vi "RSZVB Set Virtual Transform Balanced Port.vi"(0 "VISA session":refnum<visa-resource-name>, 1 "Parameter Number (1)":i32=1, 2 "Value (1.0e-12 F  (Capacitance))":dbl=1e-12 format="%^.3e", 5 "Channel (1)":i32=1, 7 "Function Type (0: Deembedding)":i32(ring) items=["Deembedding", "Embedding"], 9 "Logical Port Number (1)":i32=1, 11 "error in (no error)":errorcluster {"code" format="%.0x"}, 12 "Circuit Model (1:Serial Touchstone (.s2p) data, shunt L)":i32(ring)=1 items=["Serial Touchstone (.s2p) data, shunt L"=1, "Serial Touchstone (.s2p) data, shunt C"=2, "Shunt L, serial Touchstone (.s2p) data"=3, "Shunt C, serial Touchstone (.s2p) data"=4, "Serial Cs, shunt L"=5, "Serial Ls, shunt C"=6, "Serial Cs, shunt C"=7, "Serial Ls, shunt L"=8, "Shunt L, serial Cs"=9, "Shunt C, serial Ls"=10, "Shunt C, serial Cs"=11, "Shunt L, serial Ls"=12], 13 "Parameter Type (0: Capacitance)":i32(ring) items=["Capacitance", "Inductance", "Resistance"]) -> (4 "dup VISA session":refnum<visa-resource-name>, 15 "error out":errorcluster {"code" format="%.0x"})   [LabVIEW 2011]
doc: "This VI specifies the capacitance, inductance or resistance values C1, C2, C3, L1, L2, L3 or R1, R2, R3 in the different circuit models for balanced port deembedding/embedding.\n\nRemote-control command(s):\nCALCulate<Ch>:TRANsform:VNETworks:BALanced:DEEMbedding<Log_pt>:PARameters:C<no> STSC | SCST | CSSL | LSSC | CSSC | SLCS | SCLS | SCCS,<numeric_value>\nCALCulate<Ch>:TRANsform:VNETworks:BALanced:DEEMbedding<Log_pt>:PARameters:L<no> STSL | SLST | CSSL | LSSC | LSSL | SLCS | SCLS | SLLS,<numeric_value>\nCALCulate<Ch>:TRANsform:VNETworks:BALanced:DEEMbedding<Log_pt>:PARameters:R<no> STSL | STSC | SLST | SCST | CSSL | LSSC | CSSC | LSSL | SLCS | SCLS | SCCS | SLLS,<numeric_value>\nCALCulate<Ch>:TRANsform:VNETworks:BALanced:EMBedding<Log_pt>:PARameters:C<no> STSC | SCST | CSSL | LSSC | CSSC | SLCS | SCLS | SCCS,<numeric_value>\nCALCulate<Ch>:TRANsform:VNETworks:BALanced:EMBedding<Log_pt>:PARameters:L<no> STSL | SLST | CSSL | LSSC | LSSL | SLCS | SCLS | SLLS,<numeric_value>\nCALCulate<Ch>:TRANsform:VNETworks:BALanced:EMBedding<Log_pt>:PARameters:R<no> STSL | STSC | SLST | SCST | CSSL | LSSC | CSSC | LSSL | SLCS | SCLS | SCCS | SLLS,<numeric_value>"
uses:
  _utility/RSZVB Global Data.vi
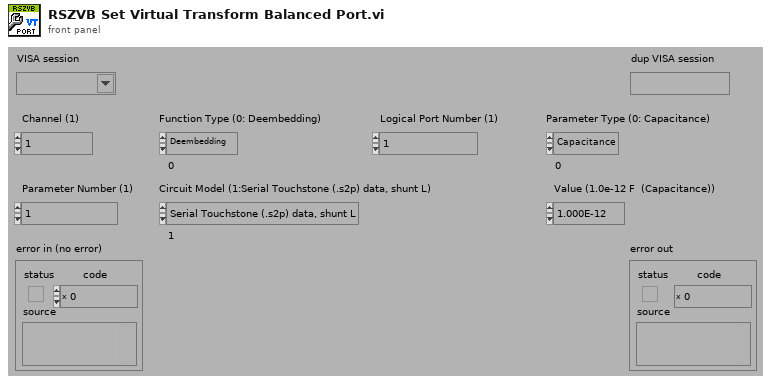
[diagram p1: front panel]
types:
  T1 = cluster{"Error Checking (T: On)":bool, "Installed Options":string[], "Data Valid?":bool, "Ports":i32, "Model":string[], "Option Checking (T: On)":bool}[]
  T2 = cluster{"Error Checking (T: On)":bool, "Installed Options":string[], "Data Valid?":bool, "Ports":i32, "Model":string[], "Option Checking (T: On)":bool}
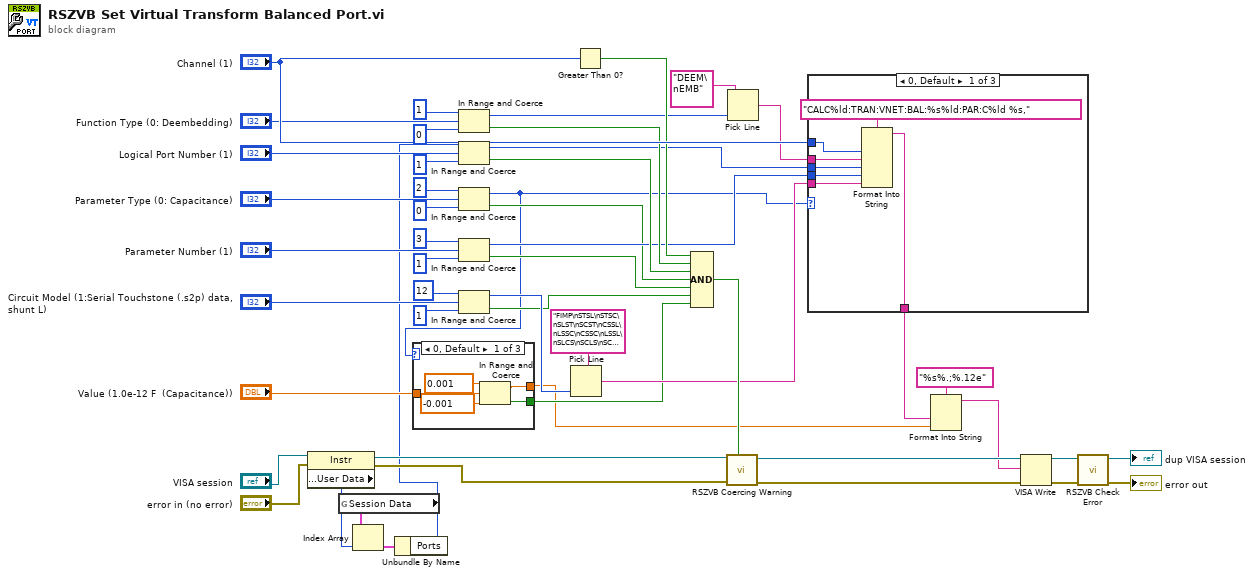
[diagram p0: block diagram]
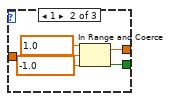
[diagram p2: hidden frame]
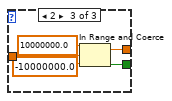
[diagram p3: hidden frame]
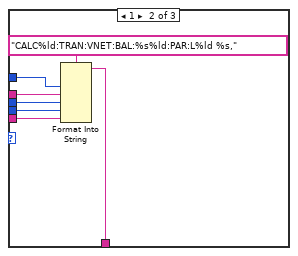
[diagram p4: hidden frame]
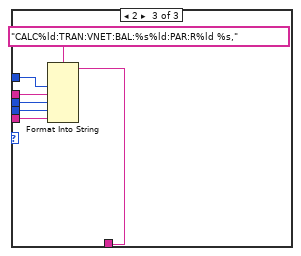
[diagram p5: hidden frame]
diagram:
  n1 = property class="Instr"(reference="VISA session", error in="error in (no error)") -> (reference out=w42:refnum<visa-resource-name>, error out=w43:errorcluster, "General Settings:User Data"=w46:u32)
  n2 = global read "RSZVB Global Data.vi" "Session Data"() -> (w45:T1)
  n3 = Index Array(array=w45, index=w46) -> (element=w44:T2)
  n4 = Unbundle By Name(w44) -> ("Ports"=w1:i32)
  n5 = In Range and Coerce(upper limit=1 ("lower limit"), x="Function Type (0: Deembedding)", lower limit=0) -> (coerced(x)=w33:i32, In Range?=w36:bool)
  n6 = In Range and Coerce(upper limit=w1, x="Logical Port Number (1)", lower limit=1) -> (coerced(x)=w35:i32, In Range?=w31:bool)
  n7 = In Range and Coerce(upper limit=2 ("lower limit"), x="Parameter Type (0: Capacitance)", lower limit=0) -> (coerced(x)=w9:i32, In Range?=w13:bool)
  n8 = case shown="0, Default" w9 {
    tunnel: [w54 w59 w64] -> w10
    tunnel: [w53 w57 w63] -> w4
    tunnel: "Value (1.0e-12 F  (Capacitance))" -> [w52 w58 w62]
    frame 0, Default {
      n9 = In Range and Coerce(upper limit=0.001, x=w52, lower limit=-0.001) -> (coerced(x)=w53:dbl, In Range?=w54:bool)
    }
    frame 1 {
      n10 = In Range and Coerce(upper limit=1.0, x=w58, lower limit=-1.0) -> (coerced(x)=w57:dbl, In Range?=w59:bool)
    }
    frame 2 {
      n11 = In Range and Coerce(upper limit=10000000.0, x=w62, lower limit=-10000000.0) -> (coerced(x)=w63:dbl, In Range?=w64:bool)
    }
  }
  n12 = In Range and Coerce(upper limit=3 ("lower limit"), x="Parameter Number (1)", lower limit=1) -> (coerced(x)=w14:i32, In Range?=w12:bool)
  n13 = In Range and Coerce(upper limit=12 ("lower limit"), x="Circuit Model (1:Serial Touchstone (.s2p) data, shunt L)", lower limit=1) -> (coerced(x)=w16:i32, In Range?=w11:bool)
  n14 = Pick Line(multi-line string="FIMP\nSTSL\nSTSC\nSLST\nSCST\nCSSL\nLSSC\nCSSC\nLSSL\nSLCS\nSCLS\nSCCS\nSLLS", line index=w16) -> (output string=w15:string)  [unwired: 1 in]
  n15 = Greater Than 0?(x="Channel (1)") -> (x > 0?=w39:bool)
  n16 = Compound Arithmetic op=AND(w39, w36, w31, w13, w12, w11, w10) -> (w38:bool)
  n17 = call "RSZVB Coercing Warning.vi"("In Range?"=w38, "error in (no error)"=w43, "VISA session"=w42) -> ("error out"=w50:errorcluster, "dup VISA session"=w51:refnum<visa-resource-name>)  [unwired: 7 in]
  n18 = Pick Line(multi-line string="DEEM\nEMB", line index=w33) -> (output string=w32:string)  [unwired: 1 in]
  n19 = case shown="0, Default" w9 {
    tunnel: "Channel (1)" -> [w72 w79 w86]
    tunnel: w35 -> [w70 w77 w84]
    tunnel: w32 -> [w71 w78 w85]
    tunnel: w15 -> [w69 w75 w82]
    tunnel: w14 -> [w68 w76 w83]
    tunnel: [w67 w74 w81] -> w5
    frame 0, Default {
      n20 = Format Into String(format string="CALC%ld:TRAN:VNET:BAL:%s%ld:PAR:C%ld %s,", w72, w71, w70, w68, w69) -> (resulting string=w67:string)  [unwired: 2 in, 1 out]
    }
    frame 1 {
      n21 = Format Into String(format string="CALC%ld:TRAN:VNET:BAL:%s%ld:PAR:L%ld %s,", w79, w78, w77, w76, w75) -> (resulting string=w74:string)  [unwired: 2 in, 1 out]
    }
    frame 2 {
      n22 = Format Into String(format string="CALC%ld:TRAN:VNET:BAL:%s%ld:PAR:R%ld %s,", w86, w85, w84, w83, w82) -> (resulting string=w81:string)  [unwired: 2 in, 1 out]
    }
  }
  n23 = Format Into String(format string="%s%.;%.12e", w5, w4) -> (resulting string=w2:string)  [unwired: 2 in, 1 out]
  n24 = VISA Write(VISA resource name=w51, write buffer=w2, error in (no error)=w50) -> (VISA resource name out=w48:refnum<visa-resource-name>, error out=w49:errorcluster)  [unwired: 1 out]
  n25 = call "RSZVB Check Error.vi"("error in (no error)"=w49, "VISA session"=w48) -> ("error out"=→"error out":errorcluster, "dup VISA session"=→"dup VISA session":refnum<visa-resource-name>)  [unwired: 8 in]
